vi "setRelativeTargetPosition.vi"(7 "MoveRelBackward?":bool=TRUE, 8 "error in":errorcluster, 9 "MoveRelDistance [µm]":dbl format="%#_13g", 10 "axis [0...2]":i32, 11 "connection ID":refnum<k5>) -> (0 "error out":errorcluster, 1 "New Target Position [µm]":dbl, 2 "axis out":u8, 3 "connection ID out":refnum<k5>)   [LabVIEW 2019, in "AMC_VIs.lvlib"]
doc: "This VI sets the target position on the corresponding axis [0...2] from the current position as a zero point.\nBy setting the input MoveRelBackward? to 'false' the target position is set to currentPosition - MoveRelDistance. If MoveRelBackward? is set to 'true' the target positoin is set to currentPosition + MoveRelDistance.\nTo start the movement to the target position, please refer to controlMove.vi."
uses:
  <userlib>/AMC300/AMC_VIs.lvlib
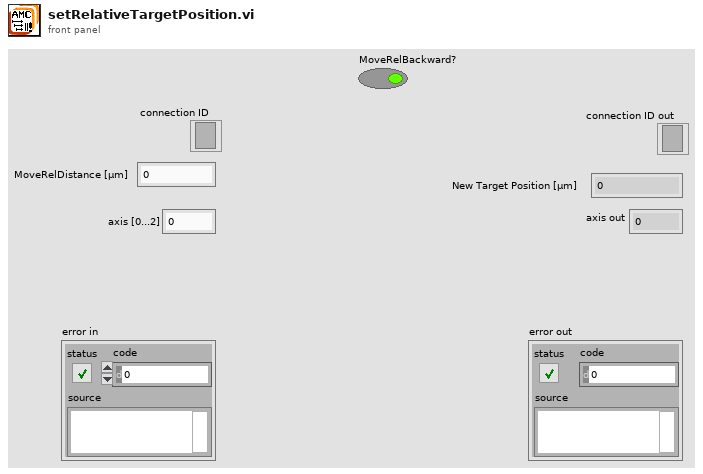
[diagram p1: front panel]
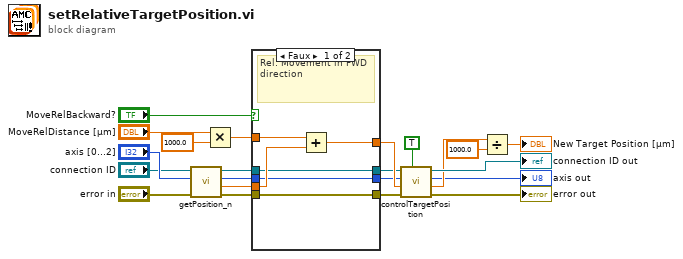
[diagram p0: block diagram]
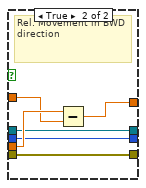
[diagram p2: hidden frame]
diagram:
  n1 = call <userlib>:"getPosition_n.vi"("error in"="error in", "axis"="axis [0...2]", "connection ID"="connection ID") -> ("error out"=w16:errorcluster, "position"=w22:dbl, "axis_out"=w19:i32, "connection ID"=w13:refnum<k5>)  [unwired: 5 in]
  n2 = Multiply(x="MoveRelDistance [µm]", y=1000.0) -> (x*y=w8:dbl)
  n3 = case shown="Faux" "MoveRelBackward?" {
    tunnel: w22 -> [w27 w34]
    tunnel: w8 -> [w28 w33]
    tunnel: [w26 w31] -> w20
    tunnel: w19 -> [w25 w32]
    tunnel: [w25 w32] -> w18
    tunnel: w16 -> [w24 w30]
    tunnel: [w24 w30] -> w15
    tunnel: w13 -> [w23 w29]
    tunnel: [w23 w29] -> w12
    frame False {
      # "Rel. Movement in FWD direction"
      n4 = Add(x=w28, y=w27) -> (x+y=w26:dbl)
    }
    frame True {
      # "Rel. Movement in BWD direction"
      n5 = Subtract(x=w34, y=w33) -> (x-y=w31:dbl)
    }
  }
  n6 = call <userlib>:"controlTargetPosition.vi"("Set"=TRUE, "error in"=w15, "Target Position [nm/µdeg]"=w20, "axis in"=w18, "connection ID"=w12) -> ("error out"=→"error out":errorcluster, "Target Position out"=w6:dbl, "axis out"=→"axis out":u8, "connection ID"=→"connection ID out":refnum<k5>)  [unwired: 3 in]
  n7 = Divide(x=w6, y=1000.0) -> (x/y=→"New Target Position [µm]":dbl)
